vi "Assemble QuadViewManager.vi"(8 "Bottom-Right View":refnum<class "IViewable.lvclass">, 9 "Bottom-Left View":refnum<class "IViewable.lvclass">, 10 "Top-Right View":refnum<class "IViewable.lvclass">, 11 "Top-Left View":refnum<class "IViewable.lvclass">) -> (3 "QuadViewManager out":refnum<class "QuadViewManager.lvclass">)   [LabVIEW 2015, in "QuadViewManager.lvlib" / "QuadViewManager.lvclass"]
doc: "<License>\nCopyright © 2017 Composed Systems, LLC | All rights reserved\nwww.composed.io\n\nAuthor: Ethan Stern <ethan.stern@composed.io>\n\nThis software is provided \"AS IS\" WITHOUT WARRANTIES, either express or implied, AND IS FOR EDUCATIONAL PURPOSES ONLY.\n</License>"
uses:
  QuadViewManager.lvclass
  Framework/IViewable/IViewable/IViewable.lvclass
  Framework/IViewManager/IViewManager Messages/Launch Nested Views Msg/Launch Nested Views Msg.lvclass/Launch Nested Views Msg.ctl
  Framework/IViewManager/IViewManager/IViewManager.lvclass/IViewManager.ctl
  Framework/IViewManager/IViewManager Messages/Launch Nested Views Msg/Pack Launch Nested Views Msg.vi
  Framework/IViewManager/IViewManager Messages/Launch Nested Views Msg/Launch Nested Views Msg.lvclass
  Framework/IViewManager/IViewManager/IViewManager.lvclass
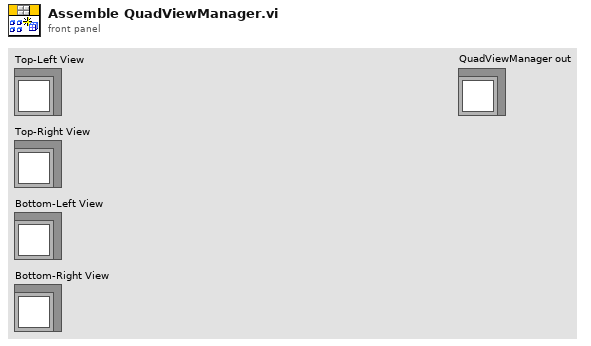
[diagram p1: front panel]
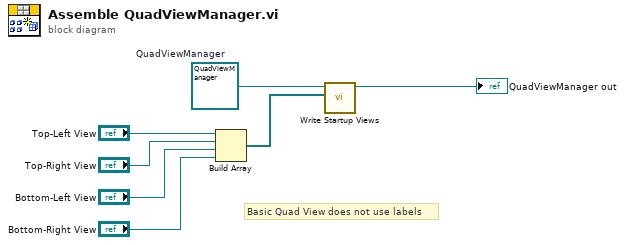
[diagram p0: block diagram]
diagram:
  w7 = refnum<class "QuadViewManager.lvclass"> refnum  # QuadViewManager
  # "Basic Quad View does not use labels"
  n1 = Build Array("Top-Left View", "Top-Right View", "Bottom-Left View", "Bottom-Right View") -> (w1:refnum<class "IViewable.lvclass">[])
  n2 = call "Write Startup Views.vi"("Startup Views"=w1, "IViewManager in"=w7) -> ("IViewManager out"=→"QuadViewManager out":refnum<class "QuadViewManager.lvclass">)  [unwired: 9 in]
